vi "Gaus Function.vi"(10 "Fit params":T1={"Amplitude"=1000.0, "Center"=694.3, "Width"=0.4, "Offset"=-500.0}, 11 "X":dbl[](array[numeric])) -> (3 "Y":dbl[](array[numeric]))   [LabVIEW 2016]
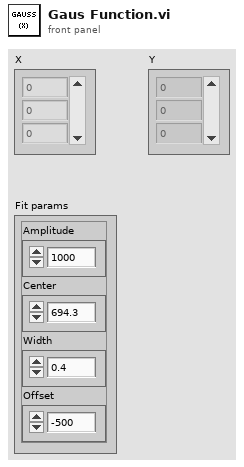
[diagram p1: front panel]
types:
  T1 = cluster{"Amplitude":dbl, "Center":dbl, "Width":dbl, "Offset":dbl}
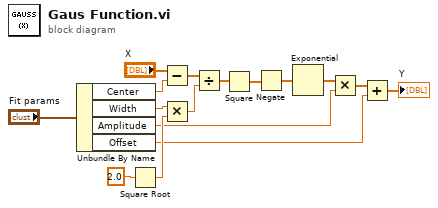
[diagram p0: block diagram]
diagram:
  n1 = Unbundle By Name("Fit params") -> ("Center"=w15:dbl, "Width"=w13:dbl, "Amplitude"=w4:dbl, "Offset"=w2:dbl)
  n2 = Square Root(x=2.0 ("y")) -> (sqrt(x)=w10:dbl)
  n3 = Subtract(x="X", y=w15) -> (x-y=w11:dbl[])
  n4 = Multiply(x=w13, y=w10) -> (x*y=w9:dbl)
  n5 = Divide(x=w11, y=w9) -> (x/y=w8:dbl[])
  n6 = Square(x=w8) -> (x^2=w7:dbl[])
  n7 = Negate(x=w7) -> (-x=w6:dbl[])
  n8 = Exponential(1:w6) -> (0:w5:dbl[])
  n9 = Multiply(x=w5, y=w4) -> (x*y=w3:dbl[])
  n10 = Add(x=w3, y=w2) -> (x+y=→"Y":dbl[])
